vi "Initialize Instrument.vi"(8 "error in (no error)":errorcluster, 10 "Reset":bool, 11 "Tektronix DPO MSO 2000 4000 in":refnum<class "Tektronix DPO MSO 2000 4000.lvclass">) -> (0 "error out":errorcluster, 3 "Tektronix DPO MSO 2000 4000 out":refnum<class "Tektronix DPO MSO 2000 4000.lvclass">)   [LabVIEW 2020, in "Tektronix DPO MSO 2000 4000.lvclass"]
uses:
  Tektronix DPO MSO 2000 4000.lvclass
  C:/Sandbox/Git_Sandbox/WiSpry Test Framework source code (LV20)/WiSpry Test Framework/Instruments/Instrument.lvclass
  Instrument.lvclass/Instrument.ctl
  Instrument.lvclass
  <instrlib>/Tektronix DPO MSO 2000 4000 Series/Tektronix DPO MSO 2000 4000 Series.lvlib
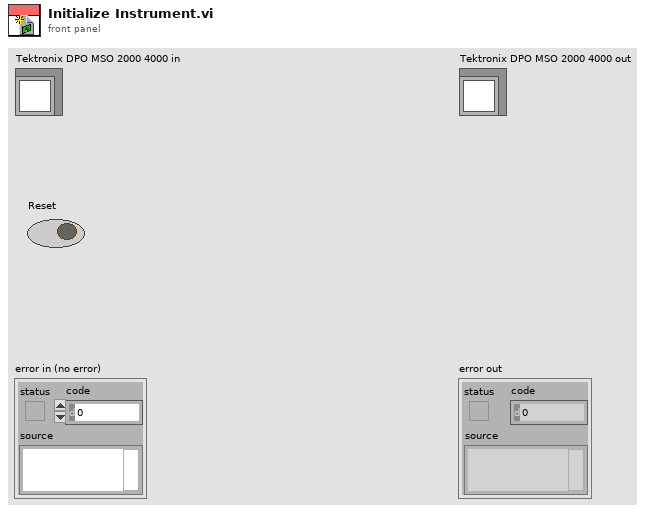
[diagram p1: front panel]
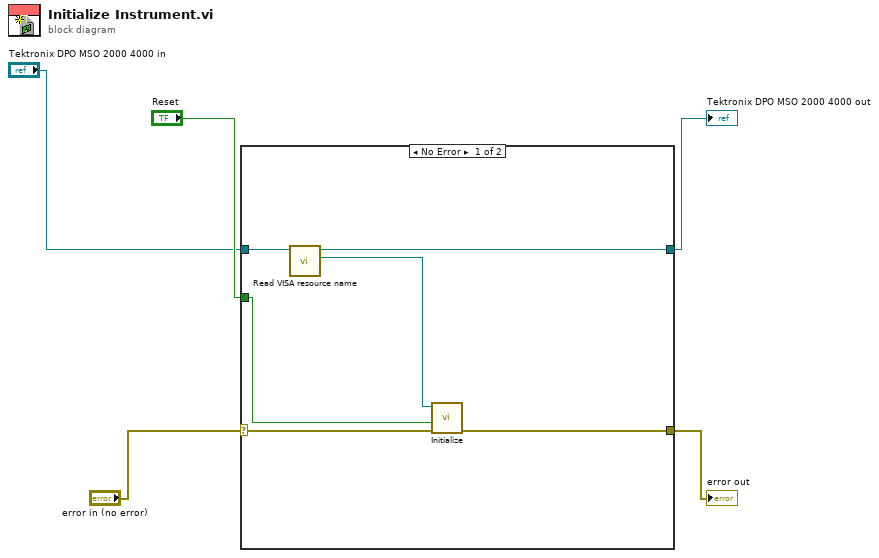
[diagram p0: block diagram]
diagram:
  n1 = case shown="No Error" "error in (no error)" {
    selector: "error in (no error)" -> [w9 w13]
    tunnel: [w8 w13] -> w1
    tunnel: [w10 w12] -> w2
    tunnel: "Tektronix DPO MSO 2000 4000 in" -> [w11 w12]
    tunnel: "Reset" -> [w6 _]
    frame No Error {
      n2 = call "Read VISA resource name.vi"("Instrument in"=w11) -> ("VISA resource name"=w7:refnum<visa-resource-name>, "Instrument out"=w10:refnum<class "Tektronix DPO MSO 2000 4000.lvclass">)  [unwired: 9 in]
      n3 = call <instrlib>:"Initialize.vi"("error in (no error)"=w9, "Reset (True)"=w6, "VISA resource name"=w7) -> ("error out"=w8:errorcluster)  [unwired: 7 in, 1 out]
    }
    frame Error {
    }
  }
  "error out" <- w1
  "Tektronix DPO MSO 2000 4000 out" <- w2
